vi "tra25cc_init.vi"(11 "com_xyz":T2) -> (0 "error IO":errorcluster, 3 "conn_xyz":T1)   [LabVIEW 2014]
uses:
  \\CL3-USR4\usr4/F103625/Scanner_v3_current/src/Stage_xyz/Dll/Newport.CONEXCC.CommandInterface.dll
  Dll/Newport.CONEXCC.CommandInterface.dll
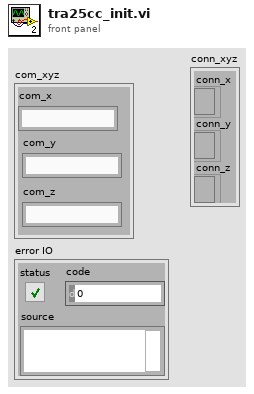
[diagram p1: front panel]
types:
  T1 = cluster{"conn_x":refnum<k24>, "conn_y":refnum<k24>, "conn_z":refnum<k24>}
  T2 = cluster{"com_x":string, "com_y":string, "com_z":string}
  T3 = cluster{"new reference":refnum<k24>, "new reference":refnum<k24>, "new reference":refnum<k24>}
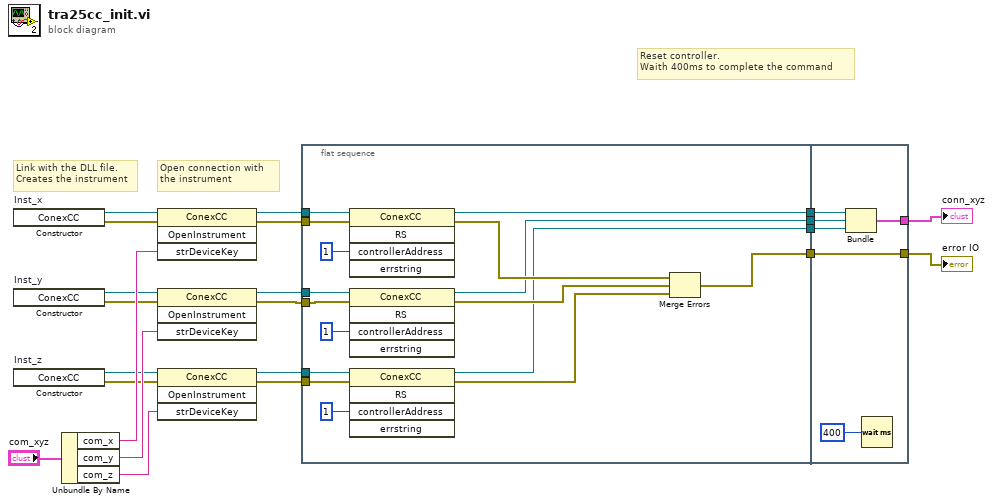
[diagram p0: block diagram]
diagram:
  # "Reset controller.\nWaith 400ms to complete the command"
  # "Link with the DLL file.\nCreates the instrument"
  # "Open connection with\nthe instrument"
  n1 = constructor on="Inst_x" class="ConexCC"() -> (reference out=w20:refnum<k24>, error out=w19:errorcluster)  [unwired: 3 in, 1 out]
  n2 = constructor on="Inst_y" class="ConexCC"() -> (reference out=w5:refnum<k24>, error out=w4:errorcluster)  [unwired: 3 in, 1 out]
  n3 = constructor on="Inst_z" class="ConexCC"() -> (reference out=w3:refnum<k24>, error out=w2:errorcluster)  [unwired: 3 in, 1 out]
  n4 = Unbundle By Name("com_xyz") -> ("com_x"=w21:string, "com_y"=w18:string, "com_z"=w17:string)
  n5 = invoke class="ConexCC" method="OpenInstrument"(reference=w20, error in=w19, "strDeviceKey"=w21) -> (reference out=w16:refnum<k24>, error out=w15:errorcluster)  [unwired: 1 in, 2 out]
  n6 = invoke class="ConexCC" method="OpenInstrument"(reference=w5, error in=w4, "strDeviceKey"=w18) -> (reference out=w12:refnum<k24>, error out=w11:errorcluster)  [unwired: 1 in, 2 out]
  n7 = invoke class="ConexCC" method="OpenInstrument"(reference=w3, error in=w2, "strDeviceKey"=w17) -> (reference out=w14:refnum<k24>, error out=w13:errorcluster)  [unwired: 1 in, 2 out]
  n8 = flat-sequence {
    tunnel: w16 -> [w38]
    tunnel: w15 -> [w37]
    tunnel: w14 -> [w33]
    tunnel: w13 -> [w32]
    tunnel: w12 -> [w31]
    tunnel: w11 -> [w30]
    tunnel: [w26] -> w10
    tunnel: [w25] -> w8
    tunnel: [w24] -> w7
    tunnel: [w23] -> w6
    tunnel: [w43] -> w9
    tunnel: w10 -> [w43]
    tunnel: w8 -> [w42]
    tunnel: [w39] -> w1
    tunnel: w7 -> [w41]
    tunnel: w6 -> [w40]
    frame #0 {
      n9 = invoke class="ConexCC" method="RS"(reference=w38, error in=w37, "controllerAddress"=1) -> (reference out=w25:refnum<k24>, error out=w29:errorcluster)  [unwired: 2 in, 3 out]
      n10 = invoke class="ConexCC" method="RS"(reference=w31, error in=w30, "controllerAddress"=1) -> (reference out=w24:refnum<k24>, error out=w28:errorcluster)  [unwired: 2 in, 3 out]
      n11 = invoke class="ConexCC" method="RS"(reference=w33, error in=w32, "controllerAddress"=1) -> (reference out=w23:refnum<k24>, error out=w27:errorcluster)  [unwired: 2 in, 3 out]
      n12 = Merge Errors(w29, w28, w27) -> (w26:errorcluster)
    }
    frame #1 {
      n13 = Bundle("new reference"=w42, "new reference"=w41, "new reference"=w40) -> (w39:T3)  [unwired: 1 in]
      n14 = Wait (ms)(milliseconds to wait=u32 400) -> ()  [unwired: 1 out]
    }
  }
  "error IO" <- w9
  "conn_xyz" <- w1
